vi "Trace Query Options.vi"(6 "Options":T2={"interpolate data (F)"=FALSE, "extrapolate to now (F)"=FALSE, "remove data breaks (F)"=FALSE, "interpolation interval (1 s)"=1.0, "maintain trending info (T)"=TRUE} {"interpolation interval (1 s)" min=0.0 format="%0.2f"}, 8 "Error In":errorcluster, 9 "Time Interval":T1 {"Stop Time" format="%<%H:%M:%S\n%Y/%m/%d>T"; "Start Time" format="%<%H:%M:%S\n%Y/%m/%d>T"}, 10 "Max Points per Trace (all)":i32=-1, 11 "BNT_DSCXtGraph in":refnum<class "BNT_DSCXtGraph.lvclass">) -> (0 "Error Out":errorcluster, 3 "BNT_DSCXtGraph out":refnum<class "BNT_DSCXtGraph.lvclass">)   [LabVIEW 2015, in "BNT_DSCXtGraph.lvlib" / "BNT_DSCXtGraph.lvclass"]
doc: "Write trace query options, query Database and update GUI."
uses:
  BNT_DSCXtGraph.lvclass
  BNT_DSCXtGraph.lvclass/BNT_DSCXtGraph.ctl
  <vilib>/ActorFramework/Actor/Actor.lvclass/Actor.ctl
  <vilib>/ActorFramework/Message Enqueuer/Message Enqueuer.lvclass/Message Enqueuer.ctl
  <vilib>/ActorFramework/Message Enqueuer/Init from Existing Queue.vi
  <vilib>/ActorFramework/Message Enqueuer/Enqueue.vi
  <vilib>/ActorFramework/Message Priority Queue/Priority Enqueue.vi
  <vilib>/ActorFramework/Message Enqueuer/Message Enqueuer.lvclass
  BNT_DSCXtGraph Messages/Read Decimated Traces Msg/Read Decimated Traces Msg.lvclass
  <vilib>/ActorFramework/Actor/Actor.lvclass
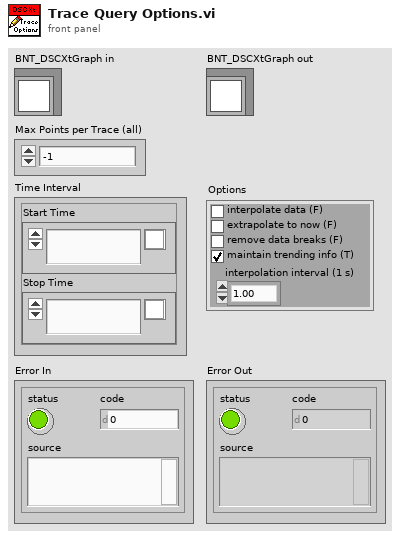
[diagram p1: front panel]
types:
  T1 = cluster{"Start Time":timestamp, "Stop Time":timestamp}
  T2 = cluster{"interpolate data (F)":bool, "extrapolate to now (F)":bool, "remove data breaks (F)":bool, "interpolation interval (1 s)":dbl, "maintain trending info (T)":bool}
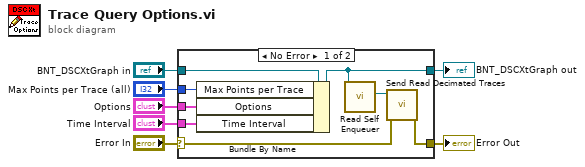
[diagram p0: block diagram]
diagram:
  n1 = case shown="No Error" "Error In" {
    selector: "Error In" -> [w9 w17]
    tunnel: [w8 w17] -> w6
    tunnel: [w11 w16] -> w4
    tunnel: "BNT_DSCXtGraph in" -> [w14 w16]
    tunnel: "Max Points per Trace (all)" -> [w15 _]
    tunnel: "Options" -> [w13 _]
    tunnel: "Time Interval" -> [w12 _]
    frame No Error {
      n2 = Bundle By Name(cluster=w14, "Max Points per Trace"=w15, "Options"=w13, "Time Interval"=w12) -> (w11:refnum<class "BNT_DSCXtGraph.lvclass">)
      n3 = call <vilib>:"Read Self Enqueuer.vi"("Actor"=w11) -> ("Self Enqueuer"=w10:refnum<class "Message Enqueuer.lvclass">)  [unwired: 10 in]
      n4 = call "Send Read Decimated Traces.vi"("error in (no error)"=w9, "Message Enqueuer"=w10) -> ("error out"=w8:errorcluster)  [unwired: 8 in, 1 out]
    }
    frame Error {
    }
  }
  "Error Out" <- w6
  "BNT_DSCXtGraph out" <- w4
